vi "利用循环结构计算从 33 到 62 之间所有整数的和.vi"() -> ()   [LabVIEW 2020]
panel:
  out "33~62累加":i32=33
  out "1~100累加":i32=33
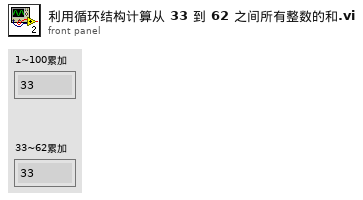
[diagram p1: front panel]
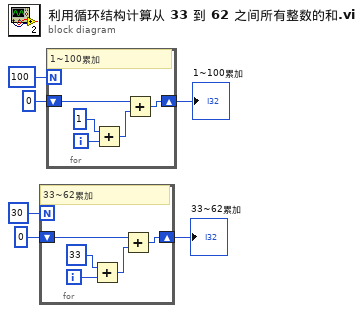
[diagram p0: block diagram]
diagram:
  n1 = for {
    N: 30 -> [_]
    shift-right: [w10] -> w3
    shift-left: 0 -> [w11]
    i -> [w8]
    # "33~62累加"
    n2 = Add(x=33, y=w8) -> (x+y=w7:i32)
    n3 = Add(x=w11, y=w7) -> (x+y=w10:i32)
  }
  "33~62累加" <- w3
  n4 = for {
    N: 100 -> [_]
    shift-right: [w15] -> w6
    shift-left: 0 -> [w16]
    i -> [w13]
    # "1~100累加"
    n5 = Add(x=1, y=w13) -> (x+y=w12:i32)
    n6 = Add(x=w16, y=w12) -> (x+y=w15:i32)
  }
  "1~100累加" <- w6
